vi "Buffer test.vi"(0 "FilePath In":path=path "/DATA/Labview Temporary Items", 1 "Buffer Size or Read#":i32, 2 "Read(0) or Write(1)":u16(ring) items=["Read", "Write", "Initialize"], 7 "Field In":dbl format="%.2f", 11 "Temperature In":dbl format="%.2f", 12 "FilePath Buffer in":path[](array[path])=[path "/DATA/Labview Temporary Items"], 13 "FIled Buffer in":dbl[](array[numeric])=[0.0] format="%.2f", 14 "Temperature Buffer in":dbl[](array[numeric])=[0.0] format="%.2f") -> (4 "FilePath out":path, 6 "Field Out":dbl format="%.2f", 8 "Temperature Out":dbl format="%.2f", 10 "Current Buffer Size":i32=200, 15 "Read Error":bool)   [LabVIEW 2020]
doc: "Write (FIFO) or retrieve (LIFO) data from the buffer.\n\nWhen write to the buffer, set the desired \"Buffer Size\" and run the VI several iterations. Notice that initially, the buffer grows to reach \"Buffer Size\" and then the input data flows from the last buffer element through to the zero element on each iteration (First In, First Out).\n\nWhen read from the buffer, set the Read# to the nth previous input data, i.e. counting reversely, with the most recent input counted as the 1st readout. If the input is out of current buffer size, an error is returned. (Last In, First Out)"
panel:
  in  "Temperature Buffer":dbl[](array[numeric])=[-1.0, -1.0, -1.0, -1.0, -1.0, -1.0, -1.0, -1.0, -1.0, -1.0, -1.0, -1.0, -1.0, -1.0, -1.0, -1.0, -1.0, -1.0, -1.0, -1.0, -1.0, -1.0, -1.0, -1.0, -1.0, -1.0, -1.0, -1.0, -1.0, -1.0, -1.0, -1.0, -1.0, -1.0, -1.0, -1.0, -1.0, -1.0, -1.0, -1.0, -1.0, -1.0, -1.0, -1.0, -1.0, -1.0, -1.0, -1.0, -1.0, -1.0, -1.0, -1.0, -1.0, -1.0, -1.0, -1.0, -1.0, -1.0, -1.0, -1.0, -1.0, -1.0, -1.0, -1.0, -1.0, -1.0, -1.0, -1.0, -1.0, -1.0, -1.0, -1.0, -1.0, -1.0, -1.0, -1.0, -1.0, -1.0, -1.0, -1.0, -1.0, -1.0, -1.0, -1.0, -1.0, -1.0, -1.0, -1.0, -1.0, -1.0, -1.0, -1.0, -1.0, -1.0, -1.0, -1.0, -1.0, -1.0, -1.0, -1.0, -1.0, -1.0, -1.0, -1.0, -1.0, -1.0, -1.0, -1.0, -1.0, -1.0, -1.0, -1.0, -1.0, -1.0, -1.0, -1.0, -1.0, -1.0, -1.0, -1.0, -1.0, -1.0, -1.0, -1.0, -1.0, -1.0, -1.0, -1.0, -1.0, -1.0, -1.0, -1.0, -1.0, -1.0, -1.0, -1.0, -1.0, -1.0, -1.0, -1.0, -1.0, -1.0, -1.0, -1.0, -1.0, -1.0, -1.0, -1.0, -1.0, -1.0, -1.0, -1.0, -1.0, -1.0, -1.0, -1.0, -1.0, -1.0, -1.0, -1.0, -1.0, -1.0, -1.0, -1.0, -1.0, -1.0, -1.0, -1.0, -1.0, -1.0, -1.0, -1.0, -1.0, -1.0, -1.0, -1.0, -1.0, -1.0, -1.0, -1.0, -1.0, -1.0, -1.0, -1.0, -1.0, -1.0, -1.0, -1.0, -1.0, -1.0, -1.0, -1.0, -1.0, -1.0, -1.0, -1.0, -1.0, -1.0, -1.0, -1.0] format="%.2f"
  in  "FIled Buffer":dbl[](array[numeric])=[24.845674253963303, 25.820873252552236, 26.831946634275432, 27.805484429325784, 28.847108492331987, 29.80821591262913, 30.431367931901146, 29.4238795700933, 28.41417787133259, 28.333962855246252, 26.403789091103846, 25.3848045654511, 24.352573903343924, 23.361452674809517, 22.34091923552048, 21.345500273188467, 20.39190491331622, 19.318773226154864, 18.291145782789922, 17.75282933001809, 16.260192541708392, 15.245460971091664, 14.257328150563565, 13.228957460079915, 12.906743744528816, 11.193036886225688, 10.19754642021276, 9.204580958436837, 8.214768508219572, 7.189551977399225, 6.192704975172958, 5.187708193247928, 4.176196848089885, 3.1911555747183797, 2.2118839269539583, 1.185521219955688, 0.17503677021148675, 0.01933369855006687, 0.039042944390315006, 0.026378295350938972, 0.8278308647225139, 1.7996470164998772, 2.82172211834191, 3.7986850369205487, 4.808379437663734, 5.808094304921966, 6.825318745962045, 7.816855667078209, 8.822675358756705, 9.80417054785586, 10.785748818107004, 11.808477843827346, 12.79682263748388, 13.825168330134716, 14.811933794042247, 15.807200774802968, 16.816611846186184, 17.776946805544426, 18.80858596434015, 19.80771370967951, 20.809332060465447, 21.81057701108441, 22.80560072729878, 23.817527037919653, 24.801684786056224, 25.816313095994857, 26.803744831521232, 27.81507987077511, 28.784535715895558, 29.803906441346587, 0.015983406771980044, 0.8337243948214059, 1.7900953104731032, 2.8017584682984316, 3.8217866734871073, 4.826199146751435, 5.828368982731004, 6.80575020906309, 7.8129931443897425, 8.812272138845596, 9.811178700099056, 10.809941479658907, 11.799343619033369, 12.802096336384245, 13.800089376277576, 14.815104283792422, 15.833527385041643, 16.820174699116983, 17.78236763209031, 18.79612074726454, 19.79220810847902, 20.80349770109635, 21.79244958103866, 22.790827203763598, 23.806442254685052, 24.78739953332719, 25.822464479222955, 26.79187289342428, 27.79432831435267, 28.8133414895027, 29.792332461853043, 0.03270413865336412, 0.8187768067367798, 1.7939255767248727, 2.777803557853667, 3.798866415240924, 4.802532644873487, 5.811365838961648, 6.797238334690081, 7.790787738694015, 8.807505823318433, 9.806180478434472, 10.821370164952796, 11.80901214403405, 12.812861777666008, 13.823286676132307, 14.794538643717258, 15.792384003457142, 16.81902020139788, 17.79858265670602, 18.832502298819747, 19.814957330854142, 20.82056261591228, 21.805569229304776, 22.806948600148854, 23.78761202536579, 24.800921286593887, 25.812034033441076, 26.81455440447704, 27.793883291737824, 28.838323620281066, 29.812628261469538, 0.061235016640850466, 0.7807385748109043, 1.792640158090274, 2.8010019108681155, 3.814540025541115, 4.819807067180232, 5.830198619671856, 6.809485779890942, 7.794921392221494, 8.787798201029217, 9.82958870729764, 10.822221987000558, 11.805937296607457, 12.816549530451969, 13.85066287972717, 14.815239820495044, 15.80855740403286, 16.800517176233082, 17.81128165744963, 18.836994688938, 19.809859304609564, 20.78963305596486, 21.787238002324404, 22.789161317781186, 23.81548160949031, 24.80005171437094, 25.80265729776752, 26.783846298307505, 27.797666355211998, 28.818214933675673, 29.820927641757184, 0.01798388374392736, 0.30433133194417095, 0.8001214150281504, 1.3243407579904027, 1.800541966127976, 2.291821166801733, 2.7732958525227764, 3.3161863546053856, 3.8066492585504257, 4.307260557462117, 4.804460277777217, 5.3131218110678535, 5.795488389311657, 6.304657736814113, 6.808578380803043, 7.280181858792316, 7.813857588132523, 8.31740539122853, 8.796009005686795, 9.33684836048933, 9.820012176653018, 10.320554008542468, 10.799456674412914, 11.299790884199968, 11.80197812940376, 12.30566527913937, 12.805083646060737, 13.327279772641145, 13.8331770277271, 14.291323430039231, 14.832818757743897, 15.299850669619563, 15.805280166673125, 16.312712597082285, 16.809878821251623, 17.30009622955457, 29.842952186020135] format="%.2f"
  in  "FilePath Buffer":path[](array[path])=[path "/DATA/980921test2/A/MyDataA+24.85T", path "/DATA/980921test2/A/MyDataA+25.82T", path "/DATA/980921test2/A/MyDataA+26.83T", path "/DATA/980921test2/A/MyDataA+27.81T", path "/DATA/980921test2/A/MyDataA+28.85T", path "/DATA/980921test2/A/MyDataA+29.81T", path "/DATA/980921test2/B/MyDataB+30.43T", path "/DATA/980921test2/B/MyDataB+29.42T", path "/DATA/980921test2/B/MyDataB+28.41T", path "/DATA/980921test2/B/MyDataB+28.33T", path "/DATA/980921test2/B/MyDataB+26.40T", path "/DATA/980921test2/B/MyDataB+25.38T", path "/DATA/980921test2/B/MyDataB+24.35T", path "/DATA/980921test2/B/MyDataB+23.36T", path "/DATA/980921test2/B/MyDataB+22.34T", path "/DATA/980921test2/B/MyDataB+21.35T", path "/DATA/980921test2/B/MyDataB+20.39T", path "/DATA/980921test2/B/MyDataB+19.32T", path "/DATA/980921test2/B/MyDataB+18.29T", path "/DATA/980921test2/B/MyDataB+17.75T", path "/DATA/980921test2/B/MyDataB+16.26T", path "/DATA/980921test2/B/MyDataB+15.25T", path "/DATA/980921test2/B/MyDataB+14.26T", path "/DATA/980921test2/B/MyDataB+13.23T", path "/DATA/980921test2/B/MyDataB+12.91T", path "/DATA/980921test2/B/MyDataB+11.19T", path "/DATA/980921test2/B/MyDataB+10.20T", path "/DATA/980921test2/B/MyDataB+09.20T", path "/DATA/980921test2/B/MyDataB+08.21T", path "/DATA/980921test2/B/MyDataB+07.19T", path "/DATA/980921test2/B/MyDataB+06.19T", path "/DATA/980921test2/B/MyDataB+05.19T", path "/DATA/980921test2/B/MyDataB+04.18T", path "/DATA/980921test2/B/MyDataB+03.19T", path "/DATA/980921test2/B/MyDataB+02.21T", path "/DATA/980921test2/B/MyDataB+01.19T", path "/DATA/980921test2/B/MyDataB+00.18T", path "", path "", path "/DATA/980921test3/A/MyDataA+00.03T", path "/DATA/980921test3/A/MyDataA+00.83T", path "/DATA/980921test3/A/MyDataA+01.80T", path "/DATA/980921test3/A/MyDataA+02.82T", path "/DATA/980921test3/A/MyDataA+03.80T", path "/DATA/980921test3/A/MyDataA+04.81T", path "/DATA/980921test3/A/MyDataA+05.81T", path "/DATA/980921test3/A/MyDataA+06.83T", path "/DATA/980921test3/A/MyDataA+07.82T", path "/DATA/980921test3/A/MyDataA+08.82T", path "/DATA/980921test3/A/MyDataA+09.80T", path "/DATA/980921test3/A/MyDataA+10.79T", path "/DATA/980921test3/A/MyDataA+11.81T", path "/DATA/980921test3/A/MyDataA+12.80T", path "/DATA/980921test3/A/MyDataA+13.83T", path "/DATA/980921test3/A/MyDataA+14.81T", path "/DATA/980921test3/A/MyDataA+15.81T", path "/DATA/980921test3/A/MyDataA+16.82T", path "/DATA/980921test3/A/MyDataA+17.78T", path "/DATA/980921test3/A/MyDataA+18.81T", path "/DATA/980921test3/A/MyDataA+19.81T", path "/DATA/980921test3/A/MyDataA+20.81T", path "/DATA/980921test3/A/MyDataA+21.81T", path "/DATA/980921test3/A/MyDataA+22.81T", path "/DATA/980921test3/A/MyDataA+23.82T", path "/DATA/980921test3/A/MyDataA+24.80T", path "/DATA/980921test3/A/MyDataA+25.82T", path "/DATA/980921test3/A/MyDataA+26.80T", path "/DATA/980921test3/A/MyDataA+27.82T", path "/DATA/980921test3/A/MyDataA+28.78T", path "/DATA/980921test3/A/MyDataA+29.80T", path "/DATA/980921test3/B/MyDataB+00.02T", path "/DATA/980921test3/B/MyDataB+00.83T", path "/DATA/980921test3/B/MyDataB+01.79T", path "/DATA/980921test3/B/MyDataB+02.80T", path "/DATA/980921test3/B/MyDataB+03.82T", path "/DATA/980921test3/B/MyDataB+04.83T", path "/DATA/980921test3/B/MyDataB+05.83T", path "/DATA/980921test3/B/MyDataB+06.81T", path "/DATA/980921test3/B/MyDataB+07.81T", path "/DATA/980921test3/B/MyDataB+08.81T", path "/DATA/980921test3/B/MyDataB+09.81T", path "/DATA/980921test3/B/MyDataB+10.81T", path "/DATA/980921test3/B/MyDataB+11.80T", path "/DATA/980921test3/B/MyDataB+12.80T", path "/DATA/980921test3/B/MyDataB+13.80T", path "/DATA/980921test3/B/MyDataB+14.82T", path "/DATA/980921test3/B/MyDataB+15.83T", path "/DATA/980921test3/B/MyDataB+16.82T", path "/DATA/980921test3/B/MyDataB+17.78T", path "/DATA/980921test3/B/MyDataB+18.80T", path "/DATA/980921test3/B/MyDataB+19.79T", path "/DATA/980921test3/B/MyDataB+20.80T", path "/DATA/980921test3/B/MyDataB+21.79T", path "/DATA/980921test3/B/MyDataB+22.79T", path "/DATA/980921test3/B/MyDataB+23.81T", path "/DATA/980921test3/B/MyDataB+24.79T", path "/DATA/980921test3/B/MyDataB+25.82T", path "/DATA/980921test3/B/MyDataB+26.79T", path "/DATA/980921test3/B/MyDataB+27.79T", path "/DATA/980921test3/B/MyDataB+28.81T", path "/DATA/980921test3/B/MyDataB+29.79T", path "/DATA/980921test3/C/MyDataC+00.03T", path "/DATA/980921test3/C/MyDataC+00.82T", path "/DATA/980921test3/C/MyDataC+01.79T", path "/DATA/980921test3/C/MyDataC+02.78T", path "/DATA/980921test3/C/MyDataC+03.80T", path "/DATA/980921test3/C/MyDataC+04.80T", path "/DATA/980921test3/C/MyDataC+05.81T", path "/DATA/980921test3/C/MyDataC+06.80T", path "/DATA/980921test3/C/MyDataC+07.79T", path "/DATA/980921test3/C/MyDataC+08.81T", path "/DATA/980921test3/C/MyDataC+09.81T", path "/DATA/980921test3/C/MyDataC+10.82T", path "/DATA/980921test3/C/MyDataC+11.81T", path "/DATA/980921test3/C/MyDataC+12.81T", path "/DATA/980921test3/C/MyDataC+13.82T", path "/DATA/980921test3/C/MyDataC+14.79T", path "/DATA/980921test3/C/MyDataC+15.79T", path "/DATA/980921test3/C/MyDataC+16.82T", path "/DATA/980921test3/C/MyDataC+17.80T", path "/DATA/980921test3/C/MyDataC+18.83T", path "/DATA/980921test3/C/MyDataC+19.81T", path "/DATA/980921test3/C/MyDataC+20.82T", path "/DATA/980921test3/C/MyDataC+21.81T", path "/DATA/980921test3/C/MyDataC+22.81T", path "/DATA/980921test3/C/MyDataC+23.79T", path "/DATA/980921test3/C/MyDataC+24.80T", path "/DATA/980921test3/C/MyDataC+25.81T", path "/DATA/980921test3/C/MyDataC+26.81T", path "/DATA/980921test3/C/MyDataC+27.79T", path "/DATA/980921test3/C/MyDataC+28.84T", path "/DATA/980921test3/C/MyDataC+29.81T", path "/DATA/980921test3/D/MyDataD+00.06T", path "/DATA/980921test3/D/MyDataD+00.78T", path "/DATA/980921test3/D/MyDataD+01.79T", path "/DATA/980921test3/D/MyDataD+02.80T", path "/DATA/980921test3/D/MyDataD+03.81T", path "/DATA/980921test3/D/MyDataD+04.82T", path "/DATA/980921test3/D/MyDataD+05.83T", path "/DATA/980921test3/D/MyDataD+06.81T", path "/DATA/980921test3/D/MyDataD+07.79T", path "/DATA/980921test3/D/MyDataD+08.79T", path "/DATA/980921test3/D/MyDataD+09.83T", path "/DATA/980921test3/D/MyDataD+10.82T", path "/DATA/980921test3/D/MyDataD+11.81T", path "/DATA/980921test3/D/MyDataD+12.82T", path "/DATA/980921test3/D/MyDataD+13.85T", path "/DATA/980921test3/D/MyDataD+14.82T", path "/DATA/980921test3/D/MyDataD+15.81T", path "/DATA/980921test3/D/MyDataD+16.80T", path "/DATA/980921test3/D/MyDataD+17.81T", path "/DATA/980921test3/D/MyDataD+18.84T", path "/DATA/980921test3/D/MyDataD+19.81T", path "/DATA/980921test3/D/MyDataD+20.79T", path "/DATA/980921test3/D/MyDataD+21.79T", path "/DATA/980921test3/D/MyDataD+22.79T", path "/DATA/980921test3/D/MyDataD+23.82T", path "/DATA/980921test3/D/MyDataD+24.80T", path "/DATA/980921test3/D/MyDataD+25.80T", path "/DATA/980921test3/D/MyDataD+26.78T", path "/DATA/980921test3/D/MyDataD+27.80T", path "/DATA/980921test3/D/MyDataD+28.82T", path "/DATA/980921test3/D/MyDataD+29.82T", path "/DATA/980921test3/E/MyDataE+00.02T", path "/DATA/980921test3/E/MyDataE+00.30T", path "/DATA/980921test3/E/MyDataE+00.80T", path "/DATA/980921test3/E/MyDataE+01.32T", path "/DATA/980921test3/E/MyDataE+01.80T", path "/DATA/980921test3/E/MyDataE+02.29T", path "/DATA/980921test3/E/MyDataE+02.77T", path "/DATA/980921test3/E/MyDataE+03.32T", path "/DATA/980921test3/E/MyDataE+03.81T", path "/DATA/980921test3/E/MyDataE+04.31T", path "/DATA/980921test3/E/MyDataE+04.80T", path "/DATA/980921test3/E/MyDataE+05.31T", path "/DATA/980921test3/E/MyDataE+05.80T", path "/DATA/980921test3/E/MyDataE+06.30T", path "/DATA/980921test3/E/MyDataE+06.81T", path "/DATA/980921test3/E/MyDataE+07.28T", path "/DATA/980921test3/E/MyDataE+07.81T", path "/DATA/980921test3/E/MyDataE+08.32T", path "/DATA/980921test3/E/MyDataE+08.80T", path "/DATA/980921test3/E/MyDataE+09.34T", path "/DATA/980921test3/E/MyDataE+09.82T", path "/DATA/980921test3/E/MyDataE+10.32T", path "/DATA/980921test3/E/MyDataE+10.80T", path "/DATA/980921test3/E/MyDataE+11.30T", path "/DATA/980921test3/E/MyDataE+11.80T", path "/DATA/980921test3/E/MyDataE+12.31T", path "/DATA/980921test3/E/MyDataE+12.81T", path "/DATA/980921test3/E/MyDataE+13.33T", path "/DATA/980921test3/E/MyDataE+13.83T", path "/DATA/980921test3/E/MyDataE+14.29T", path "/DATA/980921test3/E/MyDataE+14.83T", path "/DATA/980921test3/E/MyDataE+15.30T", path "/DATA/980921test3/E/MyDataE+15.81T", path "/DATA/980921test3/E/MyDataE+16.31T", path "/DATA/980921test3/E/MyDataE+16.81T", path "/DATA/980921test3/E/MyDataE+17.30T", path "/DATA/980921test3/F/MyDataF+29.84T"]
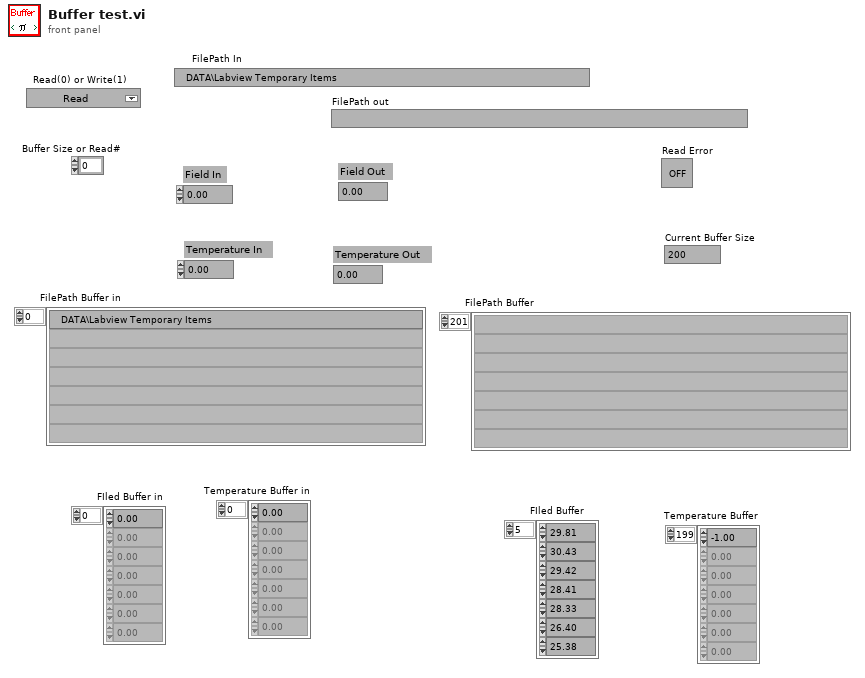
[diagram p1: front panel]
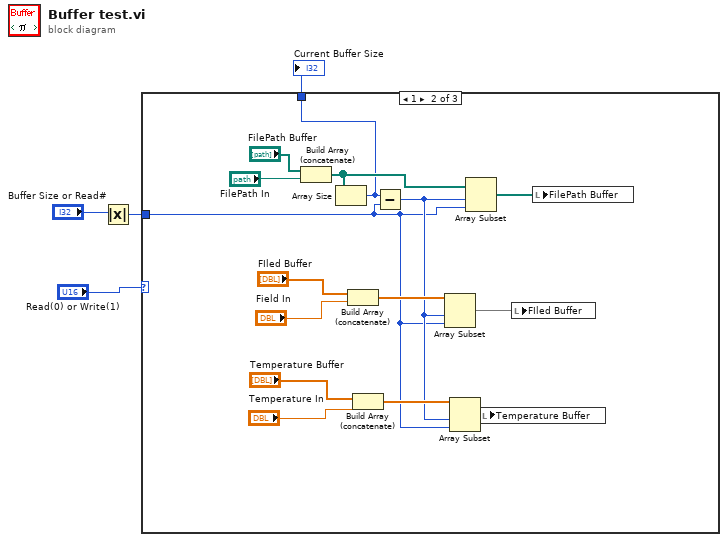
[diagram p0: block diagram]
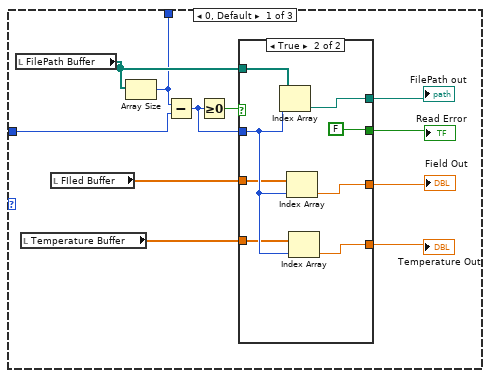
[diagram p2: hidden frame]
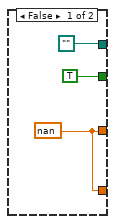
[diagram p3: hidden frame]
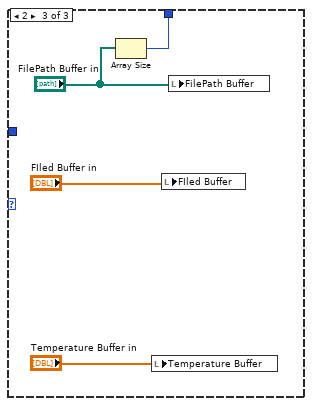
[diagram p4: hidden frame]
diagram:
  n1 = Absolute Value(x="Buffer Size or Read#") -> (abs(x)=w2:i32)
  n2 = case shown="1" "Read(0) or Write(1)" {
    tunnel: w2 -> [w14 w31 _]
    tunnel: [w11 w38 w42] -> w1
    frame 0, Default {
      n3 = local read "FilePath Buffer"() -> (w15:path[])
      n4 = local read "Temperature Buffer"() -> (w7:dbl[])
      n5 = local read "FIled Buffer"() -> (w8:dbl[])
      n6 = Array Size(array=w15) -> (size(s)=w11:i32)
      n7 = Subtract(x=w11, y=w14) -> (x-y=w12:i32)
      n8 = Greater Or Equal To 0?(x=w12) -> (x >= 0?=w13:bool)
      n9 = case shown="True" w13 {
        tunnel: w15 -> [_ w26]
        tunnel: w12 -> [_ w23]
        tunnel: [path "" w25] -> w10
        tunnel: [TRUE FALSE] -> w9
        tunnel: w8 -> [_ w22]
        tunnel: w7 -> [_ w21]
        tunnel: [w16 w20] -> w6
        tunnel: [w16 w19] -> w5
        frame False {
          w16 = nan ("sqrt(x)")
        }
        frame True {
          n10 = Index Array(array=w26, index=w23) -> (element=w25:path)
          n11 = Index Array(array=w22, index=w23) -> (element=w20:dbl)
          n12 = Index Array(array=w21, index=w23) -> (element=w19:dbl)
        }
      }
      "FilePath out" <- w10
      "Read Error" <- w9
      "Field Out" <- w6
      "Temperature Out" <- w5
    }
    frame 1 {
      n13 = Build Array (concatenate)("FilePath Buffer", "FilePath In") -> (w41:path[])
      n14 = Array Size(array=w41) -> (size(s)=w38:i32)
      n15 = Build Array (concatenate)("FIled Buffer", "Field In") -> (w34:dbl[])
      n16 = Build Array (concatenate)("Temperature Buffer", "Temperature In") -> (w33:dbl[])
      n17 = Subtract(x=w38, y=w31) -> (x-y=w32:i32)
      n18 = Array Subset(array=w34, index=w32, length=w31) -> (w28:dbl[])
      n19 = Array Subset(array=w33, index=w32, length=w31) -> (w27:dbl[])
      n20 = Array Subset(array=w41, index=w32, length=w31) -> (w39:path[])
      n21 = local write "Temperature Buffer"(w27) -> ()
      n22 = local write "FIled Buffer"(w28) -> ()
      n23 = local write "FilePath Buffer"(w39) -> ()
    }
    frame 2 {
      n24 = Array Size(array="FilePath Buffer in") -> (size(s)=w42:i32)
      n25 = local write "Temperature Buffer"("Temperature Buffer in") -> ()
      n26 = local write "FIled Buffer"("FIled Buffer in") -> ()
      n27 = local write "FilePath Buffer"("FilePath Buffer in") -> ()
    }
  }
  "Current Buffer Size" <- w1
